vi "Mutation.vi"(8 "error in (no error)":errorcluster, 11 "TSP Class in":refnum<class "TSP Class.lvclass">) -> (0 "error out":errorcluster, 3 "TSP Class out":refnum<class "TSP Class.lvclass">)   [LabVIEW 2015, in "TSP Library.lvlib" / "TSP Class.lvclass"]
uses:
  TSP Class.lvclass
  TSP Class.lvclass/TSP Class.ctl
  TSP Library.lvlib
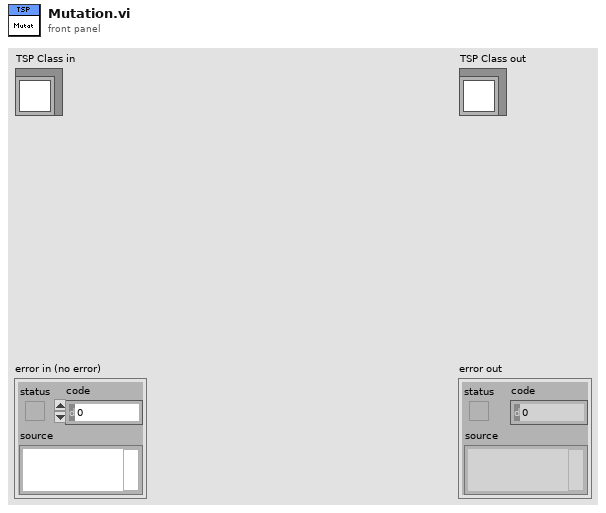
[diagram p1: front panel]
types:
  T1 = typedef "TSP Library.lvlib/Path.ctl" = cluster{"Distance":dbl, "Tour":u16[]}
  T2 = typedef "TSP Library.lvlib/Mutation.ctl" = enum16{"empty", "All v1", "All v2", "Roulette v1", "Roulette v2"}
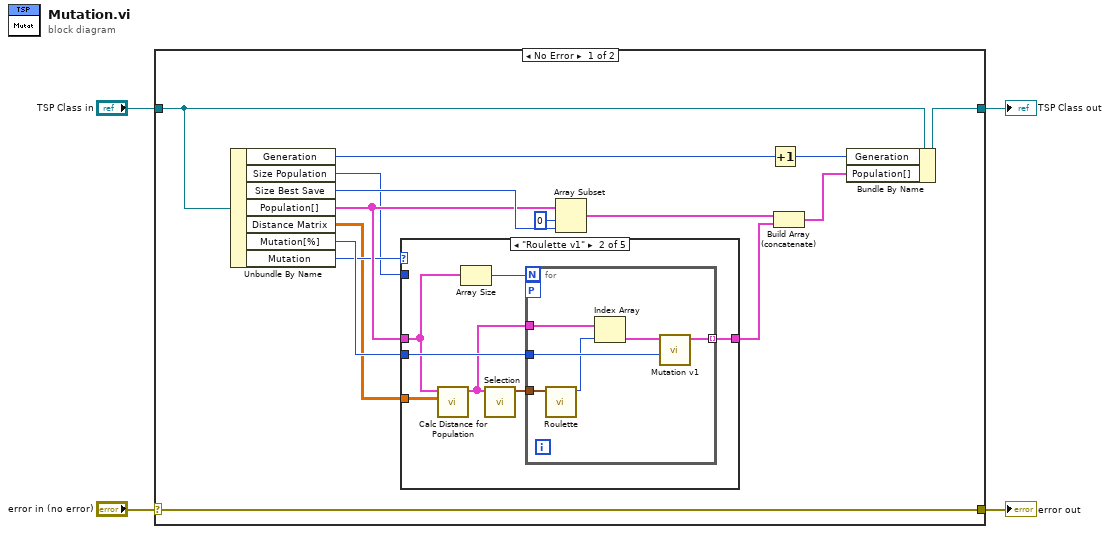
[diagram p0: block diagram]
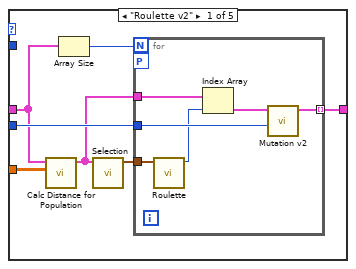
[diagram p2: hidden frame]
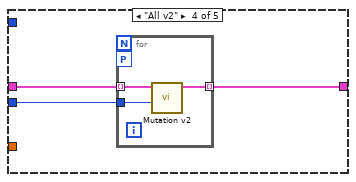
[diagram p4: hidden frame]
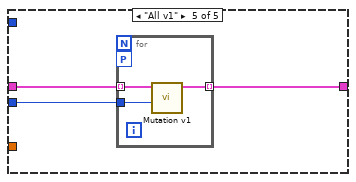
[diagram p5: hidden frame]
diagram:
  n1 = case shown="No Error" "error in (no error)" {
    selector: "error in (no error)" -> [w19 w60]
    tunnel: [w19 w60] -> w3
    tunnel: [w12 w59] -> w1
    tunnel: "TSP Class in" -> [w18 w59]
    frame No Error {
      n2 = Unbundle By Name(w18) -> ("Generation"=w11:u64, "Size Population"=w7:u16, "Size Best Save"=w16:u16, "Population[]"=w15:T1[], "Distance Matrix"=w6:dbl[][], "Mutation[%]"=w9:u8, "Mutation"=w8:T2)
      n3 = case shown="\"Roulette v1\"" w8 {
        tunnel: w15 -> [w21 w34 w46 w49 w55]
        tunnel: [w24 w37 w46 w48 w54] -> w13
        tunnel: w9 -> [w25 w38 _ w47 w53]
        tunnel: w7 -> [_ _ _ _ _]
        tunnel: w6 -> [w23 w36 _ _ _]
        frame "Roulette v2" {
          n4 = call "Calc Distance for Population.vi"("Distance Matrix"=w23, "Population[] In"=w21) -> ("Population[] Out"=w22:T1[])  [unwired: 9 in]
          n5 = Array Size(array=w21) -> (size(s)=w20:i32)
          n6 = call "Selection.vi"("Population[]"=w22) -> ("Range"=w26:cluster{dbl, dbl}[])  [unwired: 10 in]
          n7 = for {
            N: w20 -> [_]
            tunnel: w26 -> [w32]
            tunnel: w25 -> [w31]
            workers-P: _ -> [_]
            tunnel: w22 -> [w30]
            tunnel: [w27] -> w24 mode=indexing
            n8 = call "Roulette.vi"("Range"=w32) -> ("Index"=w29:i32)  [unwired: 10 in]
            n9 = Index Array(array=w30, index=w29) -> (element=w28:T1)
            n10 = call "Mutation v2.vi"("Mutation[%]"=w31, "Path In"=w28) -> ("Path Out"=w27:T1)  [unwired: 9 in]
          }
        }
        frame "Roulette v1" {
          n11 = call "Calc Distance for Population.vi"("Distance Matrix"=w36, "Population[] In"=w34) -> ("Population[] Out"=w35:T1[])  [unwired: 9 in]
          n12 = Array Size(array=w34) -> (size(s)=w33:i32)
          n13 = call "Selection.vi"("Population[]"=w35) -> ("Range"=w39:cluster{dbl, dbl}[])  [unwired: 10 in]
          n14 = for {
            N: w33 -> [_]
            tunnel: w39 -> [w45]
            tunnel: w38 -> [w44]
            workers-P: _ -> [_]
            tunnel: w35 -> [w43]
            tunnel: [w40] -> w37 mode=indexing
            n15 = call "Roulette.vi"("Range"=w45) -> ("Index"=w42:i32)  [unwired: 10 in]
            n16 = Index Array(array=w43, index=w42) -> (element=w41:T1)
            n17 = call "Mutation v1.vi"("Mutation[%]"=w44, "Path In"=w41) -> ("Path Out"=w40:T1)  [unwired: 9 in]
          }
        }
        frame "empty", Default {
        }
        frame "All v2" {
          n18 = for {
            tunnel: w49 -> [w52] mode=indexing
            tunnel: [w51] -> w48 mode=indexing
            workers-P: _ -> [_]
            tunnel: w47 -> [w50]
            n19 = call "Mutation v2.vi"("Mutation[%]"=w50, "Path In"=w52) -> ("Path Out"=w51:T1)  [unwired: 9 in]
          }
        }
        frame "All v1" {
          n20 = for {
            tunnel: w55 -> [w58] mode=indexing
            tunnel: [w57] -> w54 mode=indexing
            workers-P: _ -> [_]
            tunnel: w53 -> [w56]
            n21 = call "Mutation v1.vi"("Mutation[%]"=w56, "Path In"=w58) -> ("Path Out"=w57:T1)  [unwired: 9 in]
          }
        }
      }
      n22 = Array Subset(array=w15, index=0, length=w16) -> (w14:T1[])
      n23 = Increment(x=w11) -> (x+1=w10:u64)
      n24 = Build Array (concatenate)(w14, w13) -> (w5:T1[])
      n25 = Bundle By Name(cluster=w18, "Generation"=w10, "Population[]"=w5) -> (w12:refnum<class "TSP Class.lvclass">)
    }
    frame Error {
    }
  }
  "error out" <- w3
  "TSP Class out" <- w1
